vi "Detect 1V Cross Time.vi"(7 "CHn.Voltage":dbl[](array[numeric])) -> (8 "1V Crossing Time":dbl, 15 "error out":errorcluster)   [LabVIEW 2010]
uses:
  <vilib>/measure/mamon.llb/Trigger Detection for 1 Channel.vi
  <vilib>/measure/NI_MAPro.lvlib
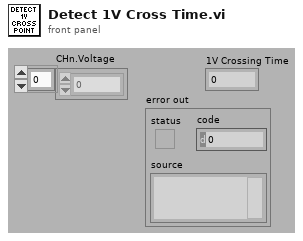
[diagram p1: front panel]
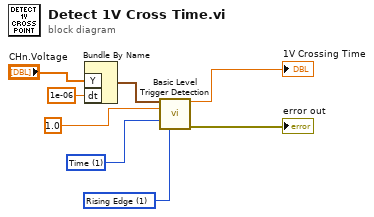
[diagram p0: block diagram]
diagram:
  w3 = u16 1 items=["Falling Edge", "Rising Edge"] ("trigger slope")
  w4 = u16 1 items=["Index", "Time"] ("location mode")
  n1 = Bundle By Name("Y"="CHn.Voltage", "dt"=1e-06) -> (w6:waveform(dbl))  [unwired: 1 in]
  n2 = call-poly <vilib>:"Basic Level Trigger Detection.vi"("signal in"=w6, "level"=1.0, "location mode"=w4, "trigger slope"=w3) -> ("trigger location"=→"1V Crossing Time":dbl, "error out"=→"error out":errorcluster)  [unwired: 9 in, 1 out]
